vi "Memory.Pointer.Write.Safe.1D.U64.vi"(8 "error in (no error)":errorcluster, 9 "count":u64 format="%d elements", 10 "buffer in":u64[](array[numeric]), 11 "pointer in":refnum<class "Memory.Pointer.lvclass">) -> (0 "error out":errorcluster, 1 "count out":u64 format="%d elements", 2 "buffer out":u64[](array[numeric]), 3 "pointer out":refnum<class "Memory.Pointer.lvclass">)   [LabVIEW 2016, in "Memory Manager.lvlib" / "Memory.Pointer.lvclass"]
doc: "Writes <b>count</b> elements from the provided <b>buffer</b> to the address specified by <b>pointer</b>.\n\n<b>Note:</b> This VI is <b>safe</b>.\n\nSafe means that this function evaluates the size parameter of <b>pointer</b> to ensure that is inbounds of allocated memory before peforming a memory read/write. Reading/writing more data to a pointer than it has allocated can corrupt or crash LabVIEW."
uses:
  Memory.Pointer.lvclass
  Memory.Pointer.lvclass/Memory.Pointer.ctl
  Accessors/Get Address.vi
  Memory.Pointer.Errors.vi
  Memory.Pointer.Errors.Buffer Underflow.vi
  Memory.Pointer.Parameter Check.Size.0D.vi
  VIs/Memory.Count to Size.Power of 2.vi
  Memory.Pointer.Errors.Null Pointer.vi
  Memory.Pointer.Errors.Create Error.vi
  Submodules/Static Error Handling/Source/Library/VIs/Static Error Handling.Source Buffer.Write.String.vi
  Submodules/Static Error Handling/Source/Library/VIs/Static Error Handling.Source Buffer.Write.Numeric.Scalar.Base10.vi
  Submodules/Static Error Handling/Source/Library/VIs/Static Error Handling.Source Buffer.Write.Numeric.Scalar.Base10 (U64).vi
  Memory.Pointer.Errors.Out of Bounds.vi
  Accessors/Get Size.vi
  Submodules/Static Error Handling/Source/Library/VIs/Static Error Handling.Error Cluster Constant.vi
  Submodules/Static Error Handling/Source/Library/VIs/Static Error Handling.Error Cluster Constant (256B).vi
  Submodules/Static Error Handling/Source/Library/VIs/Static Error Handling.Parameters.Status.Set.vi
  Submodules/Static Error Handling/Source/Library/VIs/Static Error Handling.Parameters.Code.Set.vi
  Submodules/Static Error Handling/Source/Library/VIs/Static Error Handling.Parameters.VI Source.Set.vi
  Constants/Memory.Constants.vi
  Constants/Memory.Constants.Library Name.vi
  Memory.Pointer.Errors.Get Info.vi
  Memory.Pointer.Errors.Write Pointer Size.vi
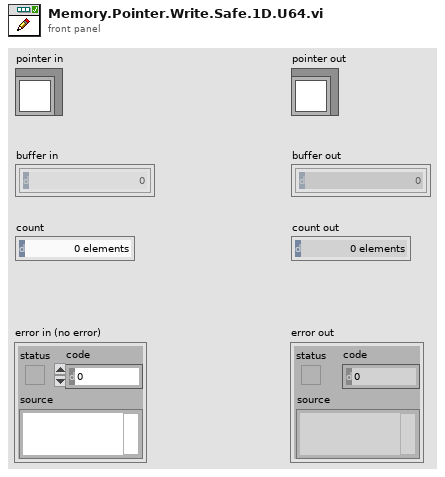
[diagram p1: front panel]
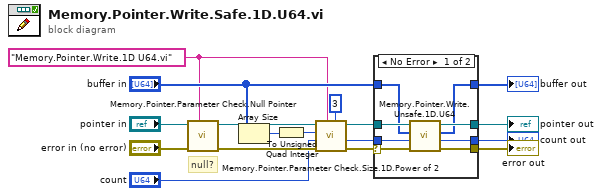
[diagram p0: block diagram]
diagram:
  w2 = "Memory.Pointer.Write.1D U64.vi" ("source vi name")
  # "null?"
  n1 = call "Memory.Pointer.Parameter Check.Null Pointer.vi"("source vi name"=w2, "error in (no error)"="error in (no error)", "Pointer in"="pointer in") -> ("error out"=w3:errorcluster, "Pointer out"=w4:refnum<class "Memory.Pointer.lvclass">)  [unwired: 7 in]
  n2 = Array Size(array="buffer in") -> (size(s)=w17:i32)
  n3 = To Unsigned Quad Integer(1:w17) -> (0:w16:u64)
  n4 = call "Memory.Pointer.Parameter Check.Size.1D.Power of 2.vi"("power of 2"=i16 3, "source vi name"=w2, "error in (no error)"=w3, "transfer count"="count", "buffer element count"=w16, "Pointer in"=w4) -> ("error out"=w15:errorcluster, "transfer count out"=w13:u64, "Pointer out"=w14:refnum<class "Memory.Pointer.lvclass">)  [unwired: 2 in, 1 out]
  n5 = case shown="No Error" w15 {
    selector: w15 -> [w25 w28]
    tunnel: w14 -> [w23 w27]
    tunnel: w13 -> [w24 w29]
    tunnel: "buffer in" -> [w19 w26]
    tunnel: [w22 w28] -> w11
    tunnel: [w21 w27] -> w7
    tunnel: [w20 w29] -> w10
    tunnel: [w18 w26] -> w8
    frame No Error {
      n6 = call "Memory.Pointer.Write.Unsafe.1D.U64.vi"("error in (no error)"=w25, "count"=w24, "buffer in"=w19, "pointer in"=w23) -> ("error out"=w22:errorcluster, "count out"=w20:u64, "buffer out"=w18:u64[], "pointer out"=w21:refnum<class "Memory.Pointer.lvclass">)  [unwired: 4 in]
    }
    frame Error {
    }
  }
  "error out" <- w11
  "pointer out" <- w7
  "buffer out" <- w8
  "count out" <- w10
